vi "rover 5.vi"() -> ()   [LabVIEW 2014]
uses:
  <vilib>/LabVIEW Interface for Arduino/Type Defs/Board Type.ctl
  <vilib>/LabVIEW Interface for Arduino/Type Defs/Connection Type.ctl
  <vilib>/LabVIEW Interface for Arduino/LabVIEW Interface for Arduino.lvlib
panel:
  out "?":dbl
  out "Numeric 3":dbl
  out "?":dbl
  out "?":dbl
  out "links voor":dbl(knob) scale=0.0..2.0
  out "links achter":dbl(knob) scale=0.0..2.0
  out "rechts voor":dbl(knob) scale=0.0..2.0
  out "rechts achter":dbl(knob) scale=0.0..2.0
  in  "links voor DIR":u8
  in  "rechts achter DIR":u8
  in  "Value (0)":u8
  in  "links achter DIR":u8
  in  "rechts voor DIR":u8
  in  "rechts achter":u8(slide) scale=0.0..255.0
  in  "rechts voor":u8(slide) scale=0.0..255.0
  in  "Voor links":u8(slide) scale=0.0..255.0
  in  "links achter":u8(slide) scale=0.0..255.0
  in  "STOP":bool
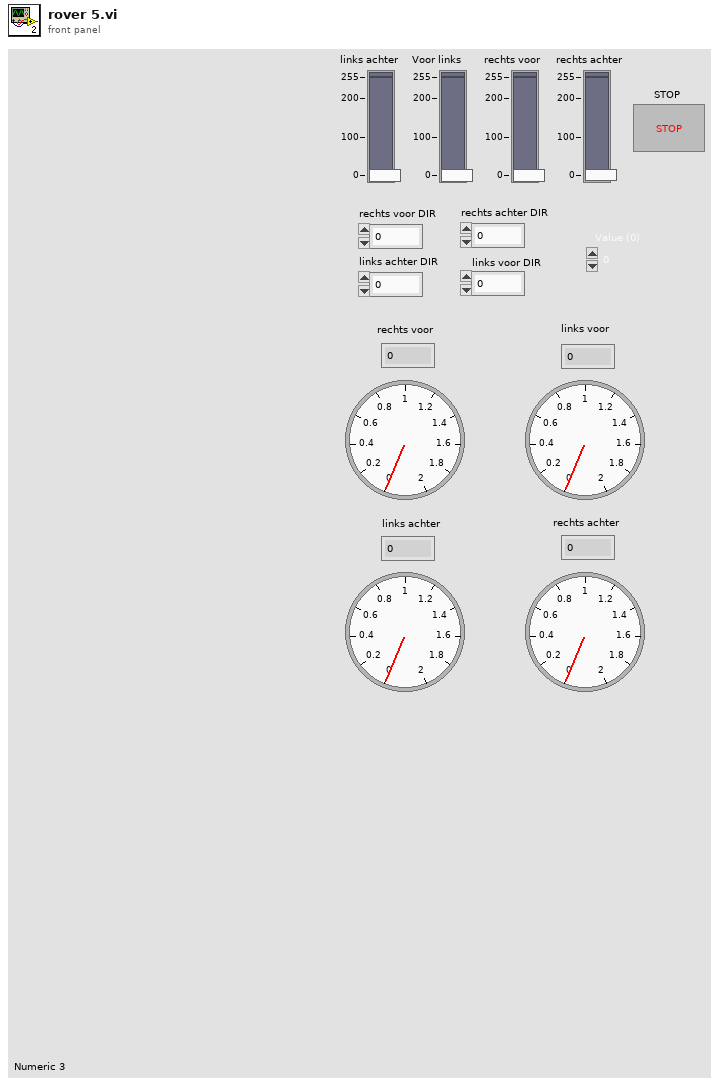
[diagram p1: front panel]
types:
  T1 = typedef "LabVIEW Interface for Arduino.lvlib/Connection Type.ctl" = enum8{"USB / Serial", "XBEE", "BlueSmirf (Bluetooth)"}
  T2 = typedef "LabVIEW Interface for Arduino.lvlib/Board Type.ctl" = enum16{"Uno", "Dimuelanove w/Atmega 328", "Mega 2560"}
  T3 = typedef "LabVIEW Interface for Arduino.lvlib/Arduino Resource.ctl" = cluster{"VISA resource":refnum<visa-resource-name>, "Board Type":T2, "Connection Type":enum8{"USB / Serial"}, "Bytes Per Packet (15)":u8}
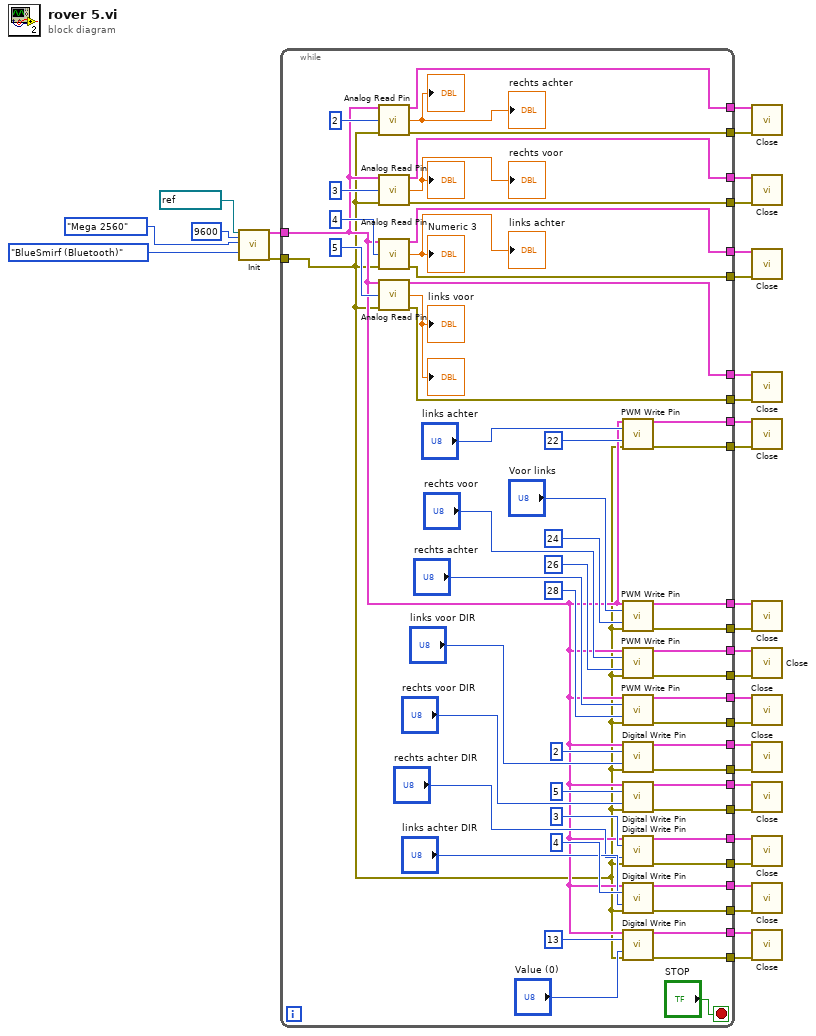
[diagram p0: block diagram]
diagram:
  n1 = call <vilib>:"Init.vi"("VISA resource"=refnum<visa-resource-name> "COM6", "Baud Rate (115200)"=u32 9600, "Board Type (Uno)"=Board_Type."Mega 2560", "Connection Type (USB/Serial)"=Connection_Type."BlueSmirf (Bluetooth)") -> ("Arduino Resource"=w32:T3, "error out"=w31:errorcluster)  [unwired: 14 in]
  n2 = while {
    tunnel: w32 -> [w34]
    tunnel: w31 -> [w33]
    tunnel: [w82] -> w26
    tunnel: [w81] -> w25
    tunnel: [w80] -> w24
    tunnel: [w78] -> w23
    tunnel: [w77] -> w22
    tunnel: [w76] -> w21
    tunnel: [w75] -> w20
    tunnel: [w79] -> w19
    tunnel: [w73] -> w18
    tunnel: [w72] -> w17
    tunnel: [w71] -> w16
    tunnel: [w70] -> w15
    tunnel: [w69] -> w14
    tunnel: [w68] -> w13
    tunnel: [w67] -> w12
    tunnel: [w62] -> w11
    tunnel: [w59] -> w10
    tunnel: [w58] -> w9
    tunnel: [w46] -> w8
    tunnel: [w45] -> w7
    tunnel: [w44] -> w6
    tunnel: [w43] -> w5
    tunnel: [w42] -> w4
    tunnel: [w41] -> w3
    tunnel: [w40] -> w2
    tunnel: [w39] -> w1
    stop <- "STOP" stop-if-true
    n3 = call <vilib>:"Analog Read Pin.vi"("Arduino Resource"=w34, "Analog Input Pin (0)"=u8 2 ("PWM Pin (3)"), "error in"=w33) -> ("Arduino Resource"=w40:T3, "Voltage"=→"rechts achter" →"?":dbl, "error out"=w39:errorcluster)  [unwired: 10 in]
    n4 = call <vilib>:"Analog Read Pin.vi"("Arduino Resource"=w34, "Analog Input Pin (0)"=u8 3 ("PWM Pin (3)"), "error in"=w33) -> ("Arduino Resource"=w42:T3, "Voltage"=→"rechts voor" →"?":dbl, "error out"=w41:errorcluster)  [unwired: 10 in]
    n5 = call <vilib>:"Analog Read Pin.vi"("Arduino Resource"=w34, "Analog Input Pin (0)"=u8 4 ("PWM Pin (3)"), "error in"=w33) -> ("Arduino Resource"=w44:T3, "Voltage"=→"links achter" →"Numeric 3":dbl, "error out"=w43:errorcluster)  [unwired: 10 in]
    n6 = call <vilib>:"Analog Read Pin.vi"("Arduino Resource"=w34, "Analog Input Pin (0)"=u8 5 ("PWM Pin (3)"), "error in"=w33) -> ("Arduino Resource"=w46:T3, "Voltage"=→"links voor" →"?":dbl, "error out"=w45:errorcluster)  [unwired: 10 in]
    n7 = call <vilib>:"PWM Write Pin.vi"("Arduino Resource"=w34, "Duty Cycle (0 - 255)"="links achter", "PWM Pin (3)"=u8 22, "error in"=w33) -> ("Arduino Resource"=w82:T3, "error out"=w81:errorcluster)  [unwired: 10 in]
    n8 = call <vilib>:"PWM Write Pin.vi"("Arduino Resource"=w34, "Duty Cycle (0 - 255)"="Voor links", "PWM Pin (3)"=u8 24, "error in"=w33) -> ("Arduino Resource"=w80:T3, "error out"=w79:errorcluster)  [unwired: 10 in]
    n9 = call <vilib>:"PWM Write Pin.vi"("Arduino Resource"=w34, "Duty Cycle (0 - 255)"="rechts voor", "PWM Pin (3)"=u8 26, "error in"=w33) -> ("Arduino Resource"=w78:T3, "error out"=w77:errorcluster)  [unwired: 10 in]
    n10 = call <vilib>:"PWM Write Pin.vi"("Arduino Resource"=w34, "Duty Cycle (0 - 255)"="rechts achter", "PWM Pin (3)"=u8 28, "error in"=w33) -> ("Arduino Resource"=w76:T3, "error out"=w75:errorcluster)  [unwired: 10 in]
    n11 = call <vilib>:"Digital Write Pin.vi"("Arduino Resource"=w34, "Digital I/O Pin (0)"=u8 2, "Value (0)"="links voor DIR", "error in"=w33) -> ("Arduino Resource"=w68:T3, "error out"=w67:errorcluster)  [unwired: 10 in]
    n12 = call <vilib>:"Digital Write Pin.vi"("Arduino Resource"=w34, "Digital I/O Pin (0)"=u8 5, "Value (0)"="rechts voor DIR", "error in"=w33) -> ("Arduino Resource"=w69:T3, "error out"=w70:errorcluster)  [unwired: 10 in]
    n13 = call <vilib>:"Digital Write Pin.vi"("Arduino Resource"=w34, "Digital I/O Pin (0)"=u8 3, "Value (0)"="rechts achter DIR", "error in"=w33) -> ("Arduino Resource"=w62:T3, "error out"=w71:errorcluster)  [unwired: 10 in]
    n14 = call <vilib>:"Digital Write Pin.vi"("Arduino Resource"=w34, "Digital I/O Pin (0)"=u8 4, "Value (0)"="links achter DIR", "error in"=w33) -> ("Arduino Resource"=w72:T3, "error out"=w73:errorcluster)  [unwired: 10 in]
    n15 = call <vilib>:"Digital Write Pin.vi"("Arduino Resource"=w34, "Digital I/O Pin (0)"=u8 13, "Value (0)"="Value (0)", "error in"=w33) -> ("Arduino Resource"=w58:T3, "error out"=w59:errorcluster)  [unwired: 10 in]
  }
  n16 = call <vilib>:"Close.vi"("Arduino Resource"=w2, "error in"=w1) -> ()  [unwired: 13 in, 1 out]
  n17 = call <vilib>:"Close.vi"("Arduino Resource"=w4, "error in"=w3) -> ()  [unwired: 13 in, 1 out]
  n18 = call <vilib>:"Close.vi"("Arduino Resource"=w6, "error in"=w5) -> ()  [unwired: 13 in, 1 out]
  n19 = call <vilib>:"Close.vi"("Arduino Resource"=w8, "error in"=w7) -> ()  [unwired: 13 in, 1 out]
  n20 = call <vilib>:"Close.vi"("Arduino Resource"=w26, "error in"=w25) -> ()  [unwired: 13 in, 1 out]
  n21 = call <vilib>:"Close.vi"("Arduino Resource"=w24, "error in"=w19) -> ()  [unwired: 13 in, 1 out]
  n22 = call <vilib>:"Close.vi"("Arduino Resource"=w23, "error in"=w22) -> ()  [unwired: 13 in, 1 out]
  n23 = call <vilib>:"Close.vi"("Arduino Resource"=w21, "error in"=w20) -> ()  [unwired: 13 in, 1 out]
  n24 = call <vilib>:"Close.vi"("Arduino Resource"=w13, "error in"=w12) -> ()  [unwired: 13 in, 1 out]
  n25 = call <vilib>:"Close.vi"("Arduino Resource"=w14, "error in"=w15) -> ()  [unwired: 13 in, 1 out]
  n26 = call <vilib>:"Close.vi"("Arduino Resource"=w11, "error in"=w16) -> ()  [unwired: 13 in, 1 out]
  n27 = call <vilib>:"Close.vi"("Arduino Resource"=w17, "error in"=w18) -> ()  [unwired: 13 in, 1 out]
  n28 = call <vilib>:"Close.vi"("Arduino Resource"=w9, "error in"=w10) -> ()  [unwired: 13 in, 1 out]
